vi "timer_functional_global.vi"(7 "State":T1, 8 "error in (no error)":errorcluster, 11 "Check Time":dbl) -> (0 "error out":errorcluster, 1 "Time Met":bool, 3 "Elapsed Time":dbl)   [LabVIEW 2011]
doc: "VI that can be used as a timer. The Start state resets the timer to the current time. The Get Time state has two features. It outputs the elapsed time from and it also checks the Check Time input and outputs a T/F if the elapsed time is > than the Check Time"
uses:
  timer_states.ctl
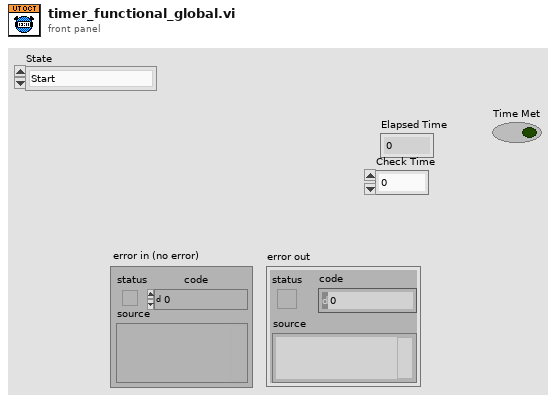
[diagram p1: front panel]
types:
  T1 = typedef "timer_states.ctl" = enum16{"Start", "Get Time"}
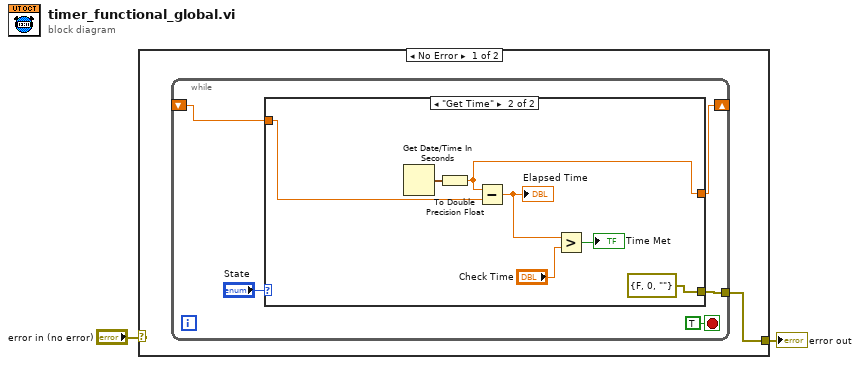
[diagram p0: block diagram]
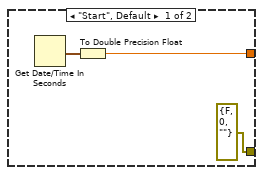
[diagram p2: hidden frame]
diagram:
  n1 = case shown="No Error" "error in (no error)" {
    selector: "error in (no error)" -> [_ w19]
    tunnel: [w3 w19] -> w1
    frame No Error {
      n2 = while {
        shift-right: [w6] -> _
        shift-left: _ -> [w5]
        tunnel: [w4] -> w3
        stop <- TRUE stop-if-true
        n3 = case shown="\"Get Time\"" "State" {
          tunnel: [w10 w15] -> w6
          tunnel: w5 -> [_ w18]
          tunnel: [errorcluster {"status"=FALSE, "code"=0, "source"=""} ("error constant") errorcluster {"status"=FALSE, "code"=0, "source"=""} ("error constant")] -> w4
          frame "Start", Default {
            n4 = Get Date/Time In Seconds() -> (seconds since 1Jan1904=w11:timestamp)
            n5 = To Double Precision Float(number=w11) -> (double precision float=w10:dbl)
          }
          frame "Get Time" {
            n6 = Get Date/Time In Seconds() -> (seconds since 1Jan1904=w17:timestamp)
            n7 = To Double Precision Float(number=w17) -> (double precision float=w15:dbl)
            n8 = Subtract(x=w15, y=w18) -> (x-y=w12:dbl)
            "Elapsed Time" <- w12
            n9 = Greater?(x=w12, y="Check Time") -> (0:→"Time Met":bool)
          }
        }
      }
    }
    frame Error {
    }
  }
  "error out" <- w1
